vi "nanocal -- nuclear schottky fit V8.vi"() -> ()   [LabVIEW 2021] (continued)
            n206 = call "replace plot - plot ref - V2.vi"("Plot ref in"=w388, "Array X IN"=w391, "Array Y IN"=w392, "plot index"=enum16{"data R(ω)", "fit R(ω)"}."data R(ω)" ("Plost: sweep window"), "cursor action"=cursor_action."write") -> ()  [unwired: 10 in, 5 out]
          }
          frame "action: replot circles" {
            n207 = local read "newton parameters"() -> (w410:T2)
            n208 = local read "parameter map"() -> (w404:map{T1, dbl})
            n209 = call "nanocal -- publish -- freq scan V2.vi"("publisher action"=publisher_action."get") -> ("data"=w408:T21)  [unwired: 7 in, 3 out]
            n210 = call "nanocal -- gradient descent -- V2.vi"("parameter tensor order IN"=w400, "data"=w408, "action"=nanocal_--_gradient_descent_--_action."peek", "newton pars"=w410, "parameter keys IN"=w409, "parameters IN"=w404) -> ("logarithmic derivatives OUT"=w405:dbl[], "ζ(ω) out"=w403:cdb[], "normalized goodness OUT"=w407:dbl)  [unwired: 2 in, 1 out]
            n211 = Absolute Value(x=w405) -> (abs(x)=w406:dbl[])
            n212 = flat-sequence {
              tunnel: w403 -> [w413]
              tunnel: w402 -> [w415]
              tunnel: "interface: update circle fit plot" ("event data") -> [w414]
              frame #0 {
                n213 = local write "R(ω) fit out"(w413) -> ()
              }
              frame #1 {
                n214 = Generate User Event(user event=w415, event data cluster=w414) -> ()  [unwired: 2 in, 2 out]
              }
            }
            n215 = local write "Goodness"(w407) -> ()
            n216 = local write "vector of dG/dlogα"(w405) -> ()
            n217 = local write "|v_i| = | dG/dlogα_i"(w406) -> ()
          }
          frame "action: plot landscape" {
            w430 = array_action."generate log range" ("action")
            n218 = property on="range one" class="Slide (strict)"() -> ("Scale.Range"=w439:T33)  [unwired: 2 in, 2 out]
            n219 = property on="range two" class="Slide (strict)"() -> ("Scale.Range"=w438:T33)  [unwired: 2 in, 2 out]
            n220 = Unbundle By Name(w439) -> ("Maximum"=w433:dbl, "Minimum"=w432:dbl)
            n221 = Unbundle By Name(w438) -> ("Maximum"=w435:dbl, "Minimum"=w434:dbl)
            n222 = local read "cursor index map"() -> (w425:map{T1, i32})
            n223 = call "array -- generate range -- V5.vi"("action"=w430, "ω points"="# points", "ω from"=w434, "ω to"=w435) -> ("ω out"=w436:dbl[])  [unwired: 7 in]
            n224 = local read "color Map"() -> (w426:map{T1, u32})
            n225 = call "array -- generate range -- V5.vi"("action"=w430, "ω points"="# points", "ω from"=w432, "ω to"=w433) -> ("ω out"=w431:dbl[])  [unwired: 7 in]
            n226 = call "nanocal -- publish -- freq scan V2.vi"("publisher action"=publisher_action."get") -> ("data"=w418:T21)  [unwired: 7 in, 3 out]
            n227 = local read "newton parameters"() -> (w420:T2)
            n228 = local read "parameter map"() -> (w417:map{T1, dbl})
            n229 = Look In Map(map=w426, key="two") -> (value=w428:u32)  [unwired: 1 in, 1 out]
            n230 = Look In Map(map=w426, key="one") -> (value=w427:u32)  [unwired: 1 in, 1 out]
            n231 = Build Array("one", "two") -> (w424:T1[])
            n232 = property on="range one" class="Slide (strict)"("Fill Color"=w427) -> ()  [unwired: 2 in, 2 out]
            n233 = property on="range two" class="Slide (strict)"("Fill Color"=w428) -> ()  [unwired: 2 in, 2 out]
            n234 = case shown="\"1d plots\", Default" "what" {
              tunnel: w417 -> [w448 w491]
              tunnel: "one" -> [_ w490]
              tunnel: w436 -> [_ w489]
              tunnel: w431 -> [w447 w488]
              tunnel: "two" -> [_ w487]
              tunnel: w426 -> [w446 _]
              tunnel: w425 -> [w445 _]
              tunnel: w424 -> [w442 _]
              tunnel: w418 -> [w443 w482]
              tunnel: w420 -> [w441 w480]
              tunnel: w419 -> [_ w481]
              tunnel: w416 -> [w440 w479]
              frame "1d plots", Default {
                n235 = control-ref of="Plot: goodness"() -> (w444:refnum<vi>)
                n236 = for {
                  tunnel: w448 -> [w456]
                  tunnel: w447 -> [w465]
                  tunnel: w442 -> [w455] mode=indexing
                  tunnel: w446 -> [w462]
                  tunnel: w445 -> [w461]
                  tunnel: w444 -> [w453]
                  tunnel: w443 -> [w452]
                  tunnel: w442 -> [w451]
                  tunnel: w441 -> [w450]
                  tunnel: w440 -> [w449]
                  n237 = for {
                    tunnel: w465 -> [w470] mode=indexing
                    tunnel: [w471] -> w467 mode=indexing
                    tunnel: [w470] -> w466 mode=indexing
                    tunnel: w456 -> [w477]
                    tunnel: w455 -> [w478]
                    tunnel: w452 -> [w476]
                    tunnel: w451 -> [w473]
                    tunnel: w450 -> [w472]
                    tunnel: w449 -> [w469]
                    n238 = Insert Into Map(map in=w477, key=w478, value=w470) -> (map out=w475:map{T1, dbl})  [unwired: 2 out]
                    n239 = call "nanocal -- gradient descent -- V2.vi"("parameter tensor order IN"=w469, "data"=w476, "action"=nanocal_--_gradient_descent_--_action."peek", "newton pars"=w472, "parameter keys IN"=w473, "parameters IN"=w475) -> ("normalized goodness OUT"=w471:dbl)  [unwired: 2 in, 3 out]
                  }
                  n240 = Look In Map(map=w456, key=w455) -> (value=w454:dbl)  [unwired: 1 in, 1 out]
                  n241 = Look In Map(map=w462, key=w455) -> (value=w457:u32)  [unwired: 1 in, 1 out]
                  n242 = Look In Map(map=w461, key=w455) -> (value=w459:i32)  [unwired: 1 in, 1 out]
                  n243 = call "replace plot - plot ref - V2.vi"("Plot ref in"=w453, "Array X IN"=w466, "Array Y IN"=w467, "plot index"=w459, "cursor action"=cursor_action."write") -> ("Plot ref out"=w464:refnum<vi>)  [unwired: 10 in, 4 out]
                  n244 = call "replace cursor - plot ref - V2.vi"("Plot ref in"=w453, "new X"=w454, "cursor index"=w459, "cursor action"=cursor_action."write", "Color Box"=w457, "cursor state"=cursor_sate."colored") -> ()  [unwired: 10 in, 4 out]
                  n245 = call "replace plot - plot ref - V2.vi"("Plot ref in"=w464, "plot index"=w459, "cursor action"=cursor_action."set plot color", "Color Box"=w457) -> ()  [unwired: 11 in, 5 out]
                }
              }
              frame "2d plots " {
                n246 = for {
                  tunnel: w491 -> [w502]
                  tunnel: w490 -> [w501]
                  tunnel: w489 -> [w500] mode=indexing
                  tunnel: w488 -> [w499]
                  tunnel: w487 -> [w498]
                  shift-right: [w496] -> w484
                  shift-left: "{ " -> [w497]
                  tunnel: w482 -> [w495]
                  tunnel: w481 -> [w494]
                  tunnel: w480 -> [w493]
                  tunnel: w479 -> [w492]
                  n247 = for {
                    tunnel: w499 -> [w511] mode=indexing
                    tunnel: w500 -> [w510]
                    tunnel: w502 -> [w524]
                    tunnel: w501 -> [w525]
                    tunnel: w498 -> [w523]
                    shift-right: [w520] -> w496
                    shift-left: w497 -> [w521]
                    tunnel: w495 -> [w508]
                    tunnel: w494 -> [w505]
                    tunnel: w493 -> [w504]
                    tunnel: w492 -> [w503]
                    w514 = " ,     "
                    w519 = i16 12 ("precision (6)")
                    n248 = Insert Into Map(map in=w524, key=w525, value=w511) -> (map out=w522:map{T1, dbl})  [unwired: 2 out]
                    n249 = Number To Fractional String(number=w511, precision (6)=w519) -> (F-format string=w518:string)  [unwired: 2 in]
                    n250 = Number To Fractional String(number=w510, precision (6)=w519) -> (F-format string=w517:string)  [unwired: 2 in]
                    n251 = Insert Into Map(map in=w522, key=w523, value=w510) -> (map out=w509:map{T1, dbl})  [unwired: 2 out]
                    n252 = call "nanocal -- gradient descent -- V2.vi"("parameter tensor order IN"=w503, "data"=w508, "action"=nanocal_--_gradient_descent_--_action."peek", "newton pars"=w504, "parameter keys IN"=w505, "parameters IN"=w509) -> ("normalized goodness OUT"=w506:dbl)  [unwired: 2 in, 3 out]
                    n253 = Number To Fractional String(number=w506, precision (6)=w519) -> (F-format string=w516:string)  [unwired: 2 in]
                    n254 = Concatenate Strings(w521, "{    ", w518, w514, w517, w514, w516, " } , ", "\r") -> (w520:string)
                  }
                }
                n255 = Concatenate Strings(w484, " }   ") -> (→"2dplots":string)
              }
            }
          }
          frame "action: gradient step" {
            (unwired) T34 {"Array "=[], "actual size"=0, "requested size"=20} ("state IN")
            w527 = 0 ("plot ind")
            n256 = local write "newton is active"(TRUE ("newton is active")) -> ()
            n257 = call "nanocal -- publish -- freq scan V2.vi"("publisher action"=publisher_action."get") -> ("data"=w532:T21)  [unwired: 7 in, 3 out]
            n258 = call "nanocal -- gradient descent -- V2.vi"("data"=w532, "action"=nanocal_--_gradient_descent_--_action."init") -> ("normalized goodness OUT"=w534:dbl)  [unwired: 6 in, 3 out]
            n259 = while {
              tunnel: w534 -> [_]
              tunnel: w530 -> [w558]
              tunnel: w531 -> [w551]
              tunnel: [w547] -> w529
              tunnel: w527 -> [_]
              shift-right: [w544] -> _
              shift-left: _ -> [w543]
              tunnel: w526 -> [w539]
              i -> [w548]
              stop <- w547 continue-if-true
              n260 = local read "newton is active"() -> (w559:bool)
              n261 = local read "factors"() -> (w562:cluster{"scaling":dbl, "what":T1}[])
              n262 = Quotient & Remainder(x=w548, y="update rate") -> (x-y*floor(x/y)=w537:i32)  [unwired: 1 out]
              n263 = Less?(x=w548, y="total # steps") -> (x < y?=w549:bool)
              n264 = local read "newton parameters"() -> (w538:T2)
              n265 = for {
                shift-right: [w601] -> w554
                shift-left: map{T1, dbl} {} ("Map IN") -> [w602]
                tunnel: w562 -> [w600] mode=indexing
                n266 = Unbundle(w600) -> ("scaling"=w598:dbl, "what"=w599:T1)
                n267 = Insert Into Map(map in=w602, key=w599, value=w598) -> (map out=w601:map{T1, dbl})  [unwired: 2 out]
              }
              n268 = local read "parameter map"() -> (w555:map{T1, dbl})
              n269 = And(x=w549, y=w559) -> (x .and. y?=w547:bool)
              n270 = case shown="0" w537 {
                tunnel: w551 -> [_ w585]
                frame 1, Default {
                }
                frame 0 {
                  n271 = Generate User Event(user event=w585, event data cluster="interface: update list from parameter map" ("event data")) -> (user event out=w584:refnum<user-event>)  [unwired: 2 in, 1 out]
                  n272 = Generate User Event(user event=w584, event data cluster="interface: update plot colors cursors" ("event data")) -> (user event out=w588:refnum<user-event>)  [unwired: 2 in, 1 out]
                  n273 = Generate User Event(user event=w588, event data cluster="interface: update circle fit plot" ("event data")) -> (user event out=w583:refnum<user-event>)  [unwired: 2 in, 1 out]
                  n274 = Generate User Event(user event=w583, event data cluster="interface: update curvature plot" ("event data")) -> ()  [unwired: 2 in, 2 out]
                }
              }
              n275 = call "nanocal -- gradient descent -- V2.vi"("parameter tensor order IN"=w539, "action"=nanocal_--_gradient_descent_--_action."step", "newton pars"=w538, "parameter keys IN"=w558, "parameters IN"=w555, "factors  IN"=w554) -> ("logarithmic derivatives OUT"=w556:dbl[], "step factors OUT"=w560:map{T1, dbl}, "ζ(ω) out"=w553:cdb[], "normalized goodness OUT"=w540:dbl)  [unwired: 2 in]
              n276 = call "aggregator - viii - real - atomic.vi"("aggregator action"=agregator_--_action."append", "requested size"="#show steps", "number"=w540, "state IN"=w543) -> ("state OUT"=w542:T34)  [unwired: 4 in, 3 out]
              n277 = case shown="0" w537 {
                tunnel: [w563 w567] -> w544
                tunnel: w542 -> [w563 w566]
                tunnel: "#show steps" -> [_ w565]
                frame 1, Default {
                }
                frame 0 {
                  n278 = call "aggregator - viii - real - atomic.vi"("aggregator action"=agregator_--_action."interpolate", "requested size"=w565, "state IN"=w566) -> ("slope"=w569:dbl, "mean"=w577:dbl, "state OUT"=w567:T34)  [unwired: 5 in, 1 out]
                  n279 = Unbundle By Name(w567) -> ("Array"=w573:dbl[], "actual size"=w576:i32)
                  n280 = for {
                    N: w565 -> [_]
                    tunnel: [w581] -> w572 mode=indexing
                    i -> [w581]
                  }
                  n281 = Decrement(x=w576) -> (x-1=w580:i32)
                  n282 = Divide(x=w580, y=2) -> (x/y=w575:dbl)
                  n283 = Subtract(x=w572, y=w575) -> (x-y=w570:dbl[])
                  n284 = Multiply(x=w570, y=w569) -> (x*y=w578:dbl[])
                  n285 = Add(x=w578, y=w577) -> (x+y=w574:dbl[])
                  n286 = Subtract(x=w573, y=w574) -> (x-y=w571:dbl[])
                  n287 = Bundle(w572, w571) -> (→"Plot: oscillations":cluster{i32[], dbl[]})  [unwired: 1 in]
                }
              }
              n288 = for {
                tunnel: w558 -> [w590] mode=indexing
                shift-right: [w594] -> _
                shift-left: w560 -> [w594]
                shift-right: [w592] -> w545
                shift-left: w555 -> [w593]
                n289 = Look In Map(map=w594, key=w590) -> (value=w591:dbl)  [unwired: 1 in, 1 out]
                n290 = in-place {
                  in-place-border: w591 -> [w596]
                  n291 = in-place-map #1(w593, w590) -> (w597:dbl)  [unwired: 1 in, 1 out]
                  n292 = Multiply(x=w596, y=w597) -> (x*y=w595:dbl)
                  n293 = in-place-map #1(w595) -> (w592:map{T1, dbl})  [unwired: 1 in, 2 out]
                }
              }
              n294 = Absolute Value(x=w556) -> (abs(x)=→"|v_i| = | dG/dlogα_i":dbl[])
              n295 = local write "R(ω) fit out"(w553) -> ()
              n296 = local write "Goodness"(w540) -> ()
              n297 = local write "vector of dG/dlogα"(w556) -> ()
              n298 = local write "parameter map"(w545) -> ()
              "current step" <- w548
            }
            n299 = local write "newton is active"(w529) -> ()
            "update  ind" <- w527
          }
          frame "action: parse string" {
            n300 = local read "String"() -> (w611:string)
            n301 = Generate User Event(user event=w603, event data cluster="interface: update list from parameter map" ("event data")) -> ()  [unwired: 2 in, 2 out]
            n302 = call "string parse mathematica assosiated array.vi"("action"=mathematica_string_map_action."parse string" ("derivative"), "String in"=w611) -> ("Map OUT"=w605:map{T1, dbl})  [unwired: 8 in, 1 out]
            n303 = Generate User Event ("action User Event")(user event=w609, event data cluster="action: update state of selectors" ("event data")) -> (user event out=w606:refnum<user-event>)  [unwired: 2 in, 1 out]
            n304 = local write "parameter map"(w605) -> ()
            n305 = Generate User Event ("action User Event")(user event=w606, event data cluster="action: replot colors" ("event data")) -> ()  [unwired: 2 in, 2 out]
          }
          frame "action: read mathematica string" {
            w621 = map{string, path} {}  # Size: 0
            w636 = map{T1, dbl} {}  # Size: 0
            w633 = set{dbl} {}  # Size: 0
            w637 = map{string, map{T1, dbl}} {}  # Size: 0
            w627 = map{string, string} {}  # Size: 0
            n306 = local read "side map to STR"() -> (w629:map{T9, string})
            n307 = local read "side map to NUM"() -> (w628:map{T9, i32})
            n308 = local read "data file parameters map"() -> (w630:map{T1, T13})
            n309 = local read "file pattern"() -> (w624:string)
            n310 = local read "folder"() -> (w625:path)
            n311 = Generate User Event(user event=w634, event data cluster="action: update enums" ("event data")) -> ()  [unwired: 2 in, 2 out]
            n312 = call "string parse mathematica list assosiated array -- V2.vi"("action"=3-lorentzian-heat-response_action."parse string" ("derivative"), "string IN"="string IN") -> ("Map OUT"=w638:map{string, map{T1, dbl}})  [unwired: 8 in, 1 out]
            n313 = call <vilib>:"Recursive File List.vi"("pattern"=w624, "Continue Recursing on Error? (F)"=TRUE, "Folder Path"=w625) -> ("All Files in Dir"=w622:path[])  [unwired: 4 in, 4 out]
            n314 = for {
              tunnel: w622 -> [w646] mode=indexing
              shift-right: [w660] -> w612
              shift-left: w638 -> [w670]
              shift-right: [w657] -> w632
              shift-left: w627 -> [w669]
              shift-right: [w656] -> w631
              shift-left: w637 -> [w665]
              shift-right: [w667] -> w616
              shift-left: w633 -> [w659]
              shift-right: [w658] -> w615
              shift-left: w633 -> [w668]
              tunnel: w636 -> [w663]
              shift-right: [w653] -> w614
              shift-left: w633 -> [w666]
              shift-right: [w655] -> w617
              shift-left: w633 -> [w664]
              tunnel: w630 -> [w662]
              shift-right: [w654] -> w619
              shift-left: w633 -> [w661]
              tunnel: w628 -> [w651]
              tunnel: w629 -> [w650]
              shift-right: [w647] -> w626
              shift-left: w621 -> [w648]
              w649 = T9[] [enum."sam", enum."ref"] items=["sam", "ref"]
              n315 = Strip Path(path=w646) -> (name=w645:string)  [unwired: 1 out]
              n316 = call "filename-manage.vi"("filename-action"=filename-action."getIDStock", "file name IN"=w645) -> ("string OUT"=w652:string)  [unwired: 7 in, 2 out]
              n317 = for {
                tunnel: w662 -> [w696]
                tunnel: w645 -> [w673]
                tunnel: w652 -> [w685]
                shift-right: [w694] -> w660
                shift-left: w670 -> [w705]
                shift-right: [w700] -> w667
                shift-left: w659 -> [w693]
                shift-right: [w692] -> w658
                shift-left: w668 -> [w701]
                shift-right: [w686] -> w653
                shift-left: w666 -> [w699]
                shift-right: [w687] -> w655
                shift-left: w664 -> [w697]
                shift-right: [w688] -> w654
                shift-left: w661 -> [w695]
                shift-right: [w689] -> w656
                shift-left: w665 -> [w698]
                shift-right: [w690] -> w657
                shift-left: w669 -> [w704]
                tunnel: w651 -> [w678]
                tunnel: w663 -> [w683]
                tunnel: w650 -> [w680]
                tunnel: w649 -> [w677] mode=indexing
                shift-right: [w674] -> w647
                shift-left: w648 -> [w675]
                tunnel: w646 -> [w672]
                # "internal key"
                n318 = Look In Map(map=w680, key=w677) -> (value=w679:string)  [unwired: 1 in, 1 out]
                n319 = Look In Map(map=w678, key=w677) -> (value=w676:i32)  [unwired: 1 in, 1 out]
                n320 = Concatenate Strings(w685, w679) -> (w684:string)
                n321 = Insert Into Map(map in=w683, key=3-lorentzian-parameters."side (S|R)", value=w676) -> (map out=w682:map{T1, dbl})  [unwired: 2 out]
                n322 = for {
                  shift-right: [w711] -> w691
                  shift-left: w682 -> [w712]
                  tunnel: w696 -> [w710] mode=indexing
                  tunnel: w673 -> [w708]
                  n323 = Unbundle(w710) -> ("key"=w709:T1, "filename-action"=w707:T13)
                  n324 = call "filename-manage.vi"("filename-action"=w707, "file name IN"=w708) -> ("number OUT"=w706:dbl)  [unwired: 7 in, 2 out]
                  n325 = Insert Into Map(map in=w712, key=w709, value=w706) -> (map out=w711:map{T1, dbl})  [unwired: 2 out]
                }
                n326 = in-place {
                  in-place-border: [w754] -> w703
                  in-place-border: w691 -> [w753]
                  n327 = in-place-map #2(w705, w684) -> (w752:map{T1, dbl}, w754:bool)  [unwired: 1 in]
                  n328 = for {
                    tunnel: w753 -> [w760] mode=indexing
                    shift-right: [w758] -> w751
                    shift-left: w752 -> [w759]
                    n329 = Unbundle(w760) -> ("key"=w757:T1, "number OUT"=w756:dbl)
                    n330 = Insert Into Map(map in=w759, key=w757, value=w756) -> (map out=w758:map{T1, dbl})  [unwired: 2 out]
                  }
                  n331 = in-place-map #2(w751, LVMapReplaceAction."Modify Entry only if found" ("action")) -> (w694:map{string, map{T1, dbl}})  [unwired: 2 out]
                }
                n332 = Not(x=w703) -> (.not. x?=w702:bool)
                n333 = case shown="True" w702 {
                  tunnel: w704 -> [w720 w750]
                  tunnel: [w720 w749] -> w690
                  tunnel: w673 -> [_ w748]
                  tunnel: w684 -> [_ w722]
                  tunnel: w701 -> [w718 w747]
                  tunnel: [w718 w746] -> w692
                  tunnel: w693 -> [w719 w745]
                  tunnel: [w719 w744] -> w700
                  tunnel: [w716 w743] -> w686
                  tunnel: w699 -> [w716 w742]
                  tunnel: w691 -> [_ w727]
                  tunnel: w698 -> [w717 w741]
                  tunnel: [w717 w740] -> w689
                  tunnel: [w715 w739] -> w687
                  tunnel: w697 -> [w715 w738]
                  tunnel: [w714 w729] -> w688
                  tunnel: w695 -> [w714 w728]
                  tunnel: w675 -> [w713 w724]
                  tunnel: [w713 w723] -> w674
                  tunnel: w672 -> [_ w721]
                  frame False {
                  }
                  frame True {
                    n334 = Look In Map(map=w727, key=3-lorentzian-parameters."set of (B|T)") -> (value=w730:dbl)  [unwired: 1 in, 1 out]
                    n335 = Look In Map(map=w727, key=3-lorentzian-parameters."side (S|R)") -> (value=w736:dbl)  [unwired: 1 in, 1 out]
                    n336 = Look In Map(map=w727, key=3-lorentzian-parameters."T (K)") -> (value=w734:dbl)  [unwired: 1 in, 1 out]
                    n337 = Look In Map(map=w727, key=3-lorentzian-parameters."B (T)") -> (value=w726:dbl)  [unwired: 1 in, 1 out]
                    n338 = Look In Map(map=w727, key=3-lorentzian-parameters."θ (deg)") -> (value=w725:dbl)  [unwired: 1 in, 1 out]
                    n339 = Insert Into Set(10:w730, 11:w728) -> (3:w729:set{dbl})  [unwired: 1 out]
                    n340 = Insert Into Set(10:w736, 11:w738) -> (3:w739:set{dbl})  [unwired: 1 out]
                    n341 = Insert Into Set(10:w734, 11:w742) -> (3:w743:set{dbl})  [unwired: 1 out]
                    n342 = Insert Into Set(10:w726, 11:w747) -> (3:w746:set{dbl})  [unwired: 1 out]
                    n343 = Insert Into Set(10:w725, 11:w745) -> (3:w744:set{dbl})  [unwired: 1 out]
                    n344 = Insert Into Map(map in=w741, key=w722, value=w727) -> (map out=w740:map{string, map{T1, dbl}})  [unwired: 2 out]
                    n345 = Insert Into Map(map in=w750, key=w722, value=w748) -> (map out=w749:map{string, string})  [unwired: 2 out]
                    n346 = Insert Into Map(map in=w724, key=w722, value=w721) -> (map out=w723:map{string, path})  [unwired: 2 out]
                  }
                }
              }
            }
            "all short filenames" <- w632
            "temps&degs" <- w631
            "mathematica thing" <- w612
            "all full filenames" <- w626
            n347 = local read "what?"() -> (w620:T6)
            n348 = in-place {
              in-place-border: w619 -> [w644]
              in-place-border: w617 -> [w643]
              in-place-border: w616 -> [w640]
              in-place-border: w615 -> [w641]
              in-place-border: w614 -> [w642]
              n349 = in-place-cluster #3(w620) -> ()  [unwired: 5 out]
              n350 = in-place-cluster #3("lookup.all set of"=w644, "lookup.all sides"=w643, "lookup.all T's"=w642, "lookup.all B's"=w641, "lookup.all θ's"=w640) -> (w618:T6)
            }
            n351 = local write "what?"(w618) -> ()
          }
          frame "action: update default values" {
            w768 = map{T1, cluster{"ζ":dbl, "ζ":dbl}[]} {}  # Size: 0
            (unwired) map{string, map{T1, dbl}} {} ("Map OUT")
            w766 = map{T1, dbl[]} {}  # Size: 0
            n352 = call "string parse mathematica list assosiated array -- V2.vi"("action"=3-lorentzian-heat-response_action."parse string" ("derivative"), "string IN"="default values string") -> ("Map OUT"=w769:map{string, map{T1, dbl}})  [unwired: 8 in, 1 out]
            n353 = Build Array (concatenate)(w764, w763, w761) -> (w762:T1[])
            n354 = for {
              tunnel: w769 -> [w795] mode=indexing
              tunnel: w762 -> [w794]
              shift-right: [w792] -> w767
              shift-left: w768 -> [w791]
              n355 = Unbundle(w795) -> ("Map"=w793:map{T1, dbl})  [unwired: 1 out]
              n356 = for {
                tunnel: w794 -> [w803] mode=indexing
                tunnel: w793 -> [w802]
                shift-right: [w797] -> w792
                shift-left: w791 -> [w796]
                # "parameter"
                # "temperatures"
                n357 = Look In Map(map=w802, key=w803) -> (value=w799:dbl)  [unwired: 1 in, 1 out]
                n358 = Look In Map(map=w796, key=w803) -> (value=w805:cluster{"ζ":dbl, "ζ":dbl}[])  [unwired: 1 in, 1 out]
                n359 = Look In Map(map=w802, key=3-lorentzian-parameters."T (K)" ("Plost: sweep window")) -> (value=w800:dbl)  [unwired: 1 in, 1 out]
                n360 = Bundle("ζ"=w800, "ζ"=w799) -> (w798:cluster{"ζ":dbl, "ζ":dbl})  [unwired: 1 in]
                n361 = Build Array (concatenate)(w805, w798) -> (w804:cluster{"ζ":dbl, "ζ":dbl}[])
                n362 = Insert Into Map(map in=w796, key=w803, value=w804) -> (map out=w797:map{T1, cluster{"ζ":dbl, "ζ":dbl}[]})  [unwired: 2 out]
              }
            }
            n363 = for {
              tunnel: w767 -> [w784] mode=indexing
              shift-right: [w781] -> w765
              shift-left: w766 -> [w780]
              # "sorted temperatures"
              # "parameter"
              # "temperatures"
              n364 = Unbundle(w784) -> ("Plost: sweep window"=w778:T1, w783:cluster{"ζ":dbl, "ζ":dbl}[])
              n365 = for {
                tunnel: w783 -> [w790] mode=indexing
                tunnel: [w789] -> w782 mode=indexing
                tunnel: [w788] -> w775 mode=indexing
                n366 = Unbundle(w790) -> ("ζ"=w789:dbl, "ζ"=w788:dbl)
              }
              n367 = call "array - sorted inexes.vi"("x"=w782) -> ("index array"=w774:i32[], "sorted array"=w776:dbl[])  [unwired: 9 in]
              n368 = Insert Into Map(map in=w780, key=3-lorentzian-parameters."T (K)", value=w776) -> (map out=w779:map{T1, dbl[]})  [unwired: 2 out]
              n369 = for {
                tunnel: w775 -> [w787]
                tunnel: w774 -> [w786] mode=indexing
                tunnel: [w785] -> w773 mode=indexing
                n370 = Index Array(array=w787, index=w786) -> (element=w785:dbl)
              }
              n371 = Insert Into Map(map in=w779, key=w778, value=w773) -> (map out=w781:map{T1, dbl[]})  [unwired: 2 out]
            }
            n372 = disable-structure shown="Disabled" {
              frame Disabled {
                # "2 3 4 0 1"
                # "2 3 4 5 6"
                # "5 6 2 3 4"
                n373 = call "array - sorted inexes.vi"() -> ()  [unwired: 10 in, 2 out]
              }
              frame Enabled {
              }
            }
            n374 = call "nanocal -- defaut parameter manager -- V1.vi"("action"=nanocal_--_defaut_parameter_manager_action--_V1."update", "internal map"=w765) -> ()  [unwired: 9 in, 1 out]
          }
          frame "action: empty string from filelist" {
            n375 = local read "file pattern"() -> (w807:string)
            n376 = local read "folder"() -> (w808:path)
            n377 = call <vilib>:"Recursive File List.vi"("pattern"=w807, "Continue Recursing on Error? (F)"=TRUE, "Folder Path"=w808) -> ("All Files in Dir"=w806:path[])  [unwired: 4 in, 4 out]
            n378 = for {
              tunnel: [w813] -> w810 mode=concatenating
              tunnel: w806 -> [w818] mode=indexing
              w816 = T9[] [enum."ref", enum."sam"] items=["sam", "ref"]
              n379 = Strip Path(path=w818) -> (name=w817:string)  [unwired: 1 out]
              n380 = local read "side map to STR"() -> (w815:map{T9, string})
              n381 = call "filename-manage.vi"("filename-action"=filename-action."getIDStock", "file name IN"=w817) -> ("string OUT"=w814:string)  [unwired: 7 in, 2 out]
              n382 = for {
                tunnel: w816 -> [w823] mode=indexing
                tunnel: w815 -> [w824]
                tunnel: w814 -> [w822]
                tunnel: [w820] -> w813 mode=indexing
                n383 = Look In Map(map=w824, key=w823) -> (value=w821:string)  [unwired: 1 in, 1 out]
                n384 = Concatenate Strings(w822, w821) -> (w820:string)
              }
            }
            n385 = call "string parse mathematica list assosiated array -- V2.vi"("action"=3-lorentzian-heat-response_action."create emty string" ("derivative"), "array of IDs"=w810) -> ("string out"=w811:string)  [unwired: 8 in, 1 out]
            n386 = local write "string OUT"(w811) -> ()
          }
          frame "action: update enums" {
            w828 = map{string, string} {}  # Size: 0
            w834 = map{i32, string} {}  # Size: 0
            # "gives a key"
            n387 = local read "what?"() -> (w826:T6)
            n388 = local read "all short filenames"() -> (w829:map{string, string})
            n389 = in-place {
              w851 = map{i32, dbl} {}  # Size: 0
              w857 = map{i32, dbl} {}  # Size: 0
              w858 = map{i32, dbl} {}  # Size: 0
              w860 = map{i32, dbl} {}  # Size: 0
              w859 = map{i32, dbl} {}  # Size: 0
              n390 = in-place-cluster #4(w826) -> ("lookup.all set of"=w845:set{dbl}, "lookup.all sides"=w844:set{dbl}, "lookup.all T's"=w843:set{dbl}, "lookup.all θ's"=w842:set{dbl}, "lookup.all B's"=w841:set{dbl})  [unwired: 5 out]
              n391 = for {
                shift-right: [w864] -> w850
                shift-left: w851 -> [w865]
                tunnel: [w862] -> w852 mode=indexing
                tunnel: w845 -> [w861] mode=indexing
                i -> [w863]
                n392 = Number To Decimal String(number=w861) -> (decimal integer string=w862:string)  [unwired: 1 in]
                n393 = Insert Into Map(map in=w865, key=w863, value=w861) -> (map out=w864:map{i32, dbl})  [unwired: 2 out]
              }
              n394 = for {
                shift-right: [w875] -> w847
                shift-left: w858 -> [w876]
                tunnel: [w873] -> w854 mode=indexing
                tunnel: w843 -> [w872] mode=indexing
                i -> [w874]
                n395 = Number To Fractional String(number=w872, precision (6)=i16 3) -> (F-format string=w873:string)  [unwired: 2 in]
                n396 = Insert Into Map(map in=w876, key=w874, value=w872) -> (map out=w875:map{i32, dbl})  [unwired: 2 out]
              }
              n397 = property on="set (1T|2B)" class="Ring (strict)"("Strings []"=w852) -> ()  [unwired: 2 in, 2 out]
              n398 = property on="T (K)" class="Ring (strict)"("Strings []"=w854) -> ()  [unwired: 2 in, 2 out]
              n399 = for {
                shift-right: [w869] -> w849
                shift-left: w857 -> [w870]
                tunnel: [w867] -> w853 mode=indexing
                tunnel: w844 -> [w866] mode=indexing
                i -> [w868]
                n400 = Number To Decimal String(number=w866) -> (decimal integer string=w867:string)  [unwired: 1 in]
                n401 = Insert Into Map(map in=w870, key=w868, value=w866) -> (map out=w869:map{i32, dbl})  [unwired: 2 out]
              }
              n402 = for {
                shift-right: [w887] -> w846
                shift-left: w859 -> [w888]
                tunnel: [w885] -> w855 mode=indexing
                tunnel: w842 -> [w884] mode=indexing
                i -> [w886]
                n403 = Number To Fractional String(number=w884, precision (6)=i16 3) -> (F-format string=w885:string)  [unwired: 2 in]
                n404 = Insert Into Map(map in=w888, key=w886, value=w884) -> (map out=w887:map{i32, dbl})  [unwired: 2 out]
              }
              n405 = property on="side (8S|4R)" class="Ring (strict)"("Strings []"=w853) -> ()  [unwired: 2 in, 2 out]
              n406 = property on="θ (∘)" class="Ring (strict)"("Strings []"=w855) -> ()  [unwired: 2 in, 2 out]
              n407 = for {
                shift-right: [w881] -> w848
                shift-left: w860 -> [w882]
                tunnel: [w879] -> w856 mode=indexing
                tunnel: w841 -> [w878] mode=indexing
                i -> [w880]
                n408 = Number To Fractional String(number=w878, precision (6)=i16 3) -> (F-format string=w879:string)  [unwired: 2 in]
                n409 = Insert Into Map(map in=w882, key=w880, value=w878) -> (map out=w881:map{i32, dbl})  [unwired: 2 out]
              }
              n410 = property on="B (T)" class="Ring (strict)"("Strings []"=w856) -> ()  [unwired: 2 in, 2 out]
              n411 = in-place-cluster #4("lookup.all set of"=w845, "lookup.all sides"=w844, "lookup.all T's"=w843, "lookup.all θ's"=w842, "lookup.all B's"=w841, "lookup.set of lookup"=w850, "lookup.side lookup"=w849, "lookup.T lookup"=w847, "lookup.B lookup"=w848, "lookup.θ lookup"=w846) -> (w825:T6)
            }
            n412 = for {
              tunnel: w829 -> [w893] mode=indexing
              shift-right: [w891] -> w827
              shift-left: w828 -> [w892]
              n413 = Unbundle(w893) -> ("event data"=w889:string, "file pattern"=w890:string)
              n414 = Insert Into Map(map in=w892, key=w890, value=w889) -> (map out=w891:map{string, string})  [unwired: 2 out]
            }
            n415 = local read "temps&degs"() -> (w833:map{string, map{T1, dbl}})
            n416 = local read "X selector"() -> (w832:T1)
            n417 = for {
              tunnel: [w902] -> w837 mode=indexing
              tunnel: [w906] -> w835 mode=indexing
              tunnel: [w903] -> w839 mode=indexing
              tunnel: w832 -> [w907]
              tunnel: w827 -> [w905] mode=indexing
              tunnel: w833 -> [w904]
              n418 = Unbundle(w905) -> (w902:string, w903:string)
              n419 = Look In Map(map=w904, key=w903) -> (value=w908:map{T1, dbl})  [unwired: 1 in, 1 out]
              n420 = Look In Map(map=w908, key=w907) -> (value=w906:dbl)  [unwired: 1 in, 1 out]
            }
            n421 = call "array - sorted inexes.vi"("x"=w835) -> ("index array"=w836:i32[])  [unwired: 9 in, 1 out]
            n422 = for {
              tunnel: w836 -> [w898] mode=indexing
              tunnel: w837 -> [w901]
              tunnel: [w900] -> w838 mode=indexing
              tunnel: w839 -> [w899]
              shift-right: [w894] -> w840
              shift-left: w834 -> [w897]
              i -> [w896]
              n423 = Index Array(array=w901, index=w898) -> (element=w900:string)
              n424 = Index Array(array=w899, index=w898) -> (element=w895:string)
              n425 = Insert Into Map(map in=w897, key=w896, value=w895) -> (map out=w894:map{i32, string})  [unwired: 2 out]
            }
            "filesnames lookup" <- w840
            n426 = property on="filenames" class="Ring (strict)"("Strings []"=w838) -> ()  [unwired: 2 in, 2 out]
            n427 = Generate User Event(user event=w830, event data cluster="action: update state of selectors" ("event data")) -> ()  [unwired: 2 in, 2 out]
            n428 = local write "what?"(w825) -> ()
          }
          frame "action: update constrained file selector" {
            w915 = map{i32, string} {}  # Size: 0
            n429 = local read "state of all selectors"() -> (w911:map{T1, map{bool, dbl}})
            n430 = local read "all short filenames"() -> (w912:map{string, string})
            n431 = local read "temps&degs"() -> (w913:map{string, map{T1, dbl}})
            n432 = for {
              tunnel: w912 -> [w925] mode=indexing
              tunnel: [w925] -> w914 mode=indexing if=w921
              shift-right: [w924] -> w910
              shift-left: w913 -> [w924]
              tunnel: w911 -> [w922]
              n433 = for {
                tunnel: [w937] -> w923 mode=indexing
                shift-right: [w932] -> _
                shift-left: w925 -> [w932]
                shift-right: [w931] -> _
                shift-left: w924 -> [w931]
                tunnel: w922 -> [w930] mode=indexing
                n434 = Unbundle(w932) -> ("event data"=w936:string)  [unwired: 1 out]
                n435 = Unbundle(w930) -> ("Plost: sweep window"=w929:T1, "map"=w928:map{bool, dbl})
                n436 = for {
                  tunnel: w928 -> [w940] mode=indexing
                  tunnel: [w939] -> w926
                  tunnel: [w938] -> w927
                  n437 = Unbundle(w940) -> ("ignore side !"=w939:bool, "number OUT"=w938:dbl)
                }
                n438 = Look In Map(map=w931, key=w936) -> (value=w935:map{T1, dbl})  [unwired: 1 in, 1 out]
                n439 = Look In Map(map=w935, key=w929) -> (value=w934:dbl)  [unwired: 1 in, 1 out]
                n440 = Equal?(x=w934, y=w927) -> (x = y?=w933:bool)
                n441 = Or(x=w926, y=w933) -> (x .or. y?=w937:bool)
              }
              n442 = And Array Elements(Boolean array=w923) -> (logical AND=w921:bool)
            }
            n443 = for {
              tunnel: [w955] -> w918 mode=indexing
              tunnel: [w953] -> w916 mode=indexing
              tunnel: [w950] -> w920 mode=indexing
              tunnel: w914 -> [w952] mode=indexing
              tunnel: w910 -> [w951]
              n444 = Unbundle(w952) -> ("event data"=w950:string, "file pattern"=w955:string)
              n445 = local read "X selector"() -> (w949:T1)
              n446 = Look In Map(map=w951, key=w950) -> (value=w954:map{T1, dbl})  [unwired: 1 in, 1 out]
              n447 = Look In Map(map=w954, key=w949) -> (value=w953:dbl)  [unwired: 1 in, 1 out]
            }
            n448 = call "array - sorted inexes.vi"("x"=w916) -> ("index array"=w917:i32[])  [unwired: 9 in, 1 out]
            n449 = for {
              tunnel: w917 -> [w945] mode=indexing
              tunnel: w918 -> [w948]
              tunnel: [w947] -> w919 mode=indexing
              tunnel: w920 -> [w946]
              shift-right: [w941] -> w909
              shift-left: w915 -> [w944]
              i -> [w943]
              n450 = Index Array(array=w948, index=w945) -> (element=w947:string)
              n451 = Index Array(array=w946, index=w945) -> (element=w942:string)
              n452 = Insert Into Map(map in=w944, key=w943, value=w942) -> (map out=w941:map{i32, string})  [unwired: 2 out]
            }
            "constrained filename lookup" <- w909
            n453 = property on="selection :|\\" class="Ring (strict)"("Strings []"=w919) -> ()  [unwired: 2 in, 2 out]
          }
          frame "action: constrained filenames select" {
            (unwired) 1
            n454 = local read "constrained filename lookup"() -> (w958:map{i32, string})
            n455 = local read "selection :|\\"() -> (w959:u16)
            n456 = local read "all full filenames"() -> (w960:map{string, path})
            n457 = Look In Map(map=w958, key=w959) -> (value=w961:string)  [unwired: 1 in, 1 out]
            n458 = Look In Map(map=w960, key=w961) -> (value=w962:path)  [unwired: 1 in, 1 out]
            n459 = local write "Read from file"(w962) -> ()
            n460 = Generate User Event(user event=w957, event data cluster="action: read from file" ("event data")) -> ()  [unwired: 2 in, 2 out]
          }
          frame "action: write mathematica string" {
            n461 = local read "mathematica thing"() -> (w967:map{string, map{T1, dbl}})
            n462 = local read "folder"() -> (w966:path)
            n463 = Build Path(base path=w966, name or relative path="temporarystring.txt") -> (appended path=w965:path)
            n464 = call "string parse mathematica list assosiated array -- V2.vi"("action"=3-lorentzian-heat-response_action."create string" ("derivative"), "Map IN"=w967) -> ("string out"=w963:string)  [unwired: 8 in, 1 out]
            "string OUT" <- w963
            n465 = Write to Text File(file (use dialog)=w965, text=w963) -> ()  [unwired: 2 in, 3 out]
          }
          frame "action: replot colors" {
            # "all -- including kappa0"
            n466 = local read "new selector names"() -> (w985:map{T1, map{T14, string}})
            n467 = local read "state of all selectors string"() -> (w980:string)
            n468 = local read "X selector"() -> (w981:T1)
            n469 = local read "state of all selectors"() -> (w992:map{T1, map{bool, dbl}})
            n470 = local read "mathematica thing"() -> (w993:map{string, map{T1, dbl}})
            n471 = Look In Map(map=w985, key=w981) -> (value=w984:map{T14, string})  [unwired: 1 in, 1 out]
            n472 = Look In Map(map=w984, key=nameformattingitem."nameL") -> (value=w982:string)  [unwired: 1 in, 1 out]
            n473 = Build Array (concatenate)(w973, w971, w970, w969) -> (w972:T1[])
            n474 = Concatenate Strings(w980, w982) -> (w991:string)
            n475 = for {
              tunnel: w993 -> [w1014]
              tunnel: w981 -> [w1009]
              tunnel: w972 -> [w997] mode=indexing
              tunnel: w992 -> [w1010]
              tunnel: w985 -> [w1001]
              shift-right: [w1005] -> w979
              shift-left: w991 -> [w1008]
              tunnel: w980 -> [w1006]
              tunnel: [w1002] -> w978 mode=indexing
              n476 = for {
                tunnel: w1014 -> [w1028] mode=indexing
                tunnel: w997 -> [w1027]
                tunnel: [w1026] -> w1013 mode=indexing if=w1020
                tunnel: [w1025] -> w1012 mode=indexing if=w1020
                tunnel: w1009 -> [w1024]
                tunnel: w1010 -> [w1023]
                n477 = Unbundle(w1028) -> ("Map"=w1022:map{T1, dbl})  [unwired: 1 out]
                n478 = for {
                  tunnel: w1023 -> [w1037] mode=indexing
                  tunnel: w1022 -> [w1036]
                  tunnel: [w1034] -> w1021 mode=indexing
                  n479 = Unbundle(w1037) -> ("Plost: sweep window"=w1035:T1, "map"=w1033:map{bool, dbl})
                  n480 = for {
                    tunnel: w1033 -> [w1040] mode=indexing
                    tunnel: [w1039] -> w1030
                    tunnel: [w1038] -> w1031
                    n481 = Unbundle(w1040) -> ("ignore side !"=w1039:bool, "number OUT"=w1038:dbl)
                  }
                  n482 = Look In Map(map=w1036, key=w1035) -> (value=w1032:dbl)  [unwired: 1 in, 1 out]
                  n483 = Equal?(x=w1032, y=w1031) -> (x = y?=w1029:bool)
                  n484 = Or(x=w1030, y=w1029) -> (x .or. y?=w1034:bool)
                }
                n485 = Look In Map(map=w1022, key=w1024) -> (value=w1026:dbl)  [unwired: 1 in, 1 out]
                n486 = Look In Map(map=w1022, key=w1027) -> (value=w1025:dbl)  [unwired: 1 in, 1 out]
                n487 = And Array Elements(Boolean array=w1021) -> (logical AND=w1020:bool)
              }
              n488 = Look In Map(map=w1001, key=w997) -> (value=w999:map{T14, string})  [unwired: 1 in, 1 out]
              n489 = Look In Map(map=w999, key=nameformattingitem."nameL") -> (value=w998:string)  [unwired: 1 in, 1 out]
              n490 = call <vilib>:"Space Constant.vi"() -> ("String"=w1007:string)
              n491 = Concatenate Strings(w1008, w1007, w1006, w998) -> (w1005:string)
              n492 = call "array - sorted inexes.vi"("x"=w1013) -> ("index array"=w1011:i32[])  [unwired: 9 in, 1 out]
              n493 = for {
                tunnel: w1013 -> [w1019]
                tunnel: w1012 -> [w1018]
                tunnel: w1011 -> [w1015] mode=indexing
                tunnel: [w1017] -> w1004 mode=indexing
                tunnel: [w1016] -> w1003 mode=indexing
                n494 = Index Array(array=w1019, index=w1015) -> (element=w1017:dbl)
                n495 = Index Array(array=w1018, index=w1015) -> (element=w1016:dbl)
              }
              n496 = Bundle(w1004, w1003) -> (w1002:cluster{dbl[], dbl[]})  [unwired: 1 in]
            }
            n497 = local read "folder"() -> (w990:path)
            n498 = Concatenate Strings("plotstring", w980, ".dat") -> (w986:string)
            n499 = Build Path(base path=w990, name or relative path=w986) -> (appended path=w989:path)
            n500 = call "nanocal -- plotstring file manage.vi"("Enum"=nanocal_--_plotstring_file_action."generate plotstring thing", "all data"=w978, "header line"=w979) -> ("plotstring thing"=w976:string)  [unwired: 8 in]
            n501 = flat-sequence {
              tunnel: w978 -> [w994]
              tunnel: w975 -> [w996]
              tunnel: "interface: replot colors plot" ("event data") -> [w995]
              frame #0 {
                "color data" <- w994
              }
              frame #1 {
                n502 = Generate User Event(user event=w996, event data cluster=w995) -> ()  [unwired: 2 in, 2 out]
              }
            }
            n503 = Write to Text File(file (use dialog)=w989, text=w976) -> ()  [unwired: 2 in, 3 out]
